vi "Periodic Tasks.vi"(8 "error in (no error)":errorcluster) -> ()   [LabVIEW 2019]
doc: "This VI runs in parallel to other tasks. It can contain as many user-defined periodic loops as you need. These can carry out PID or other sorts of timed response."
uses:
  <vilib>/Rock Robotics/WPI/ThirdParty/PhotonVisionLib/SubVI/PhotonVision_Globals.vi
  <vilib>/Rock Robotics/Network Tables/NT Write Number.vi
  <vilib>/Rock Robotics/Network Tables/NT Write Boolean.vi
  <vilib>/Rock Robotics/WPI/ThirdParty/PhotonVisionLib/PhotonVisionLib.lvlib
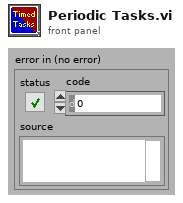
[diagram p1: front panel]
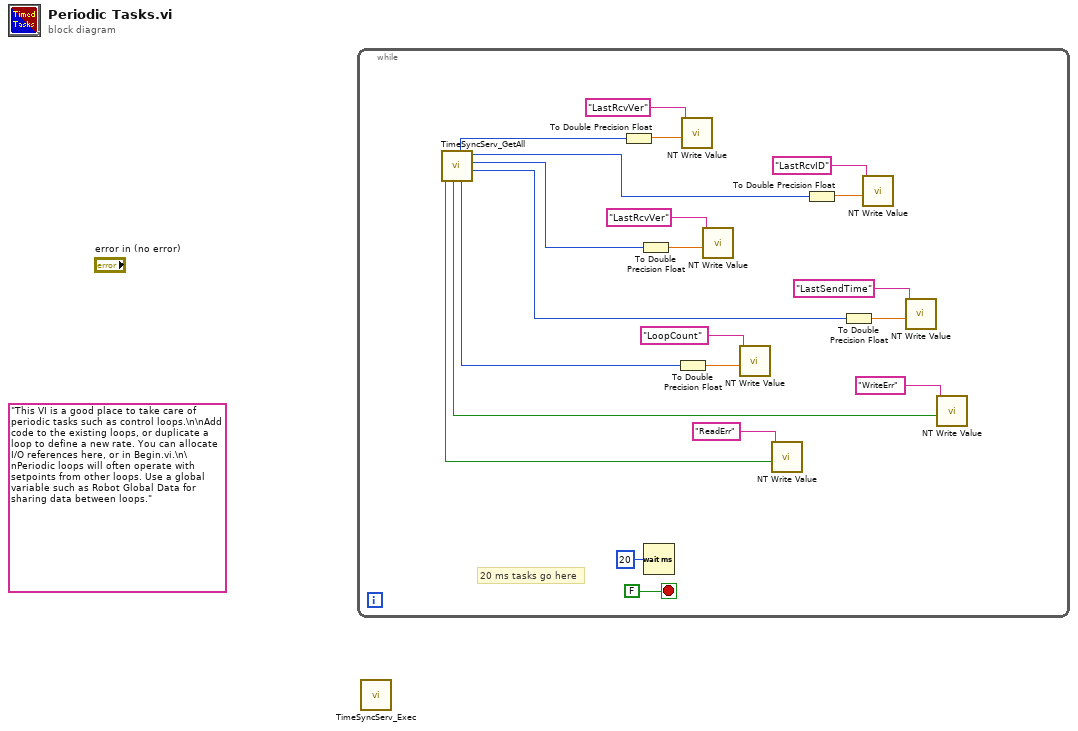
[diagram p0: block diagram]
diagram:
  (unwired) "This VI is a good place to take care of periodic tasks such as control loops.\n\nAdd code to the existing loops, or duplicate a loop to define a new rate. You can allocate I/O references here, or in Begin.vi.\n\nPeriodic loops will often operate with setpoints from other loops. Use a global variable such as Robot Global Data for sharing data between loops."
  n1 = while {
    stop <- FALSE stop-if-true
    # "20 ms tasks go here"
    n2 = call <vilib>:"TimeSyncServ_GetAll.vi"() -> ("PV_TimeSyncLastSentTime"=w8:i64, "PV_TimeSyncLastRcvTim"=w11:i64, "PV_TimeSyncLastRcvId"=w12:i8, "PV_TimeSyncLoopCount"=w5:i32, "PV_TimeSyncLastRcvVer"=w13:i8, "PV_TimeSyncServWriteErr"=w3:bool, "PV_TimeSyncServReadErr"=w1:bool)  [unwired: 4 in, 1 out]
    n3 = To Double Precision Float(number=w13) -> (double precision float=w15:dbl)
    n4 = To Double Precision Float(number=w11) -> (double precision float=w16:dbl)
    n5 = Wait (ms)(milliseconds to wait=u32 20) -> ()  [unwired: 1 out]
    n6 = To Double Precision Float(number=w5) -> (double precision float=w6:dbl)
    n7 = call-poly <vilib>:"NT Write Value.vi"("Numeric"=w15, "Name"="LastRcvVer") -> ()  [unwired: 9 in, 1 out]
    n8 = call-poly <vilib>:"NT Write Value.vi"("Numeric"=w16, "Name"="LastRcvVer") -> ()  [unwired: 9 in, 1 out]
    n9 = call-poly <vilib>:"NT Write Value.vi"("Numeric"=w6, "Name"="LoopCount") -> ()  [unwired: 9 in, 1 out]
    n10 = call-poly <vilib>:"NT Write Value.vi"("Boolean"=w1, "Name"="ReadErr") -> ()  [unwired: 9 in, 1 out]
    n11 = To Double Precision Float(number=w12) -> (double precision float=w14:dbl)
    n12 = To Double Precision Float(number=w8) -> (double precision float=w9:dbl)
    n13 = call-poly <vilib>:"NT Write Value.vi"("Numeric"=w14, "Name"="LastRcvID") -> ()  [unwired: 9 in, 1 out]
    n14 = call-poly <vilib>:"NT Write Value.vi"("Numeric"=w9, "Name"="LastSendTime") -> ()  [unwired: 9 in, 1 out]
    n15 = call-poly <vilib>:"NT Write Value.vi"("Boolean"=w3, "Name"="WriteErr") -> ()  [unwired: 9 in, 1 out]
  }
  n16 = call <vilib>:"TimeSyncServ_Exec.vi"() -> ()  [unwired: 12 in]
